vi "lib Hours Minutes Second to Degrees.vi"(8 "error in (no error)":errorcluster, 11 "Right Ascension cluster":T1) -> (0 "error out":errorcluster, 3 "Angle":dbl format="%#.8g")   [LabVIEW 2021]
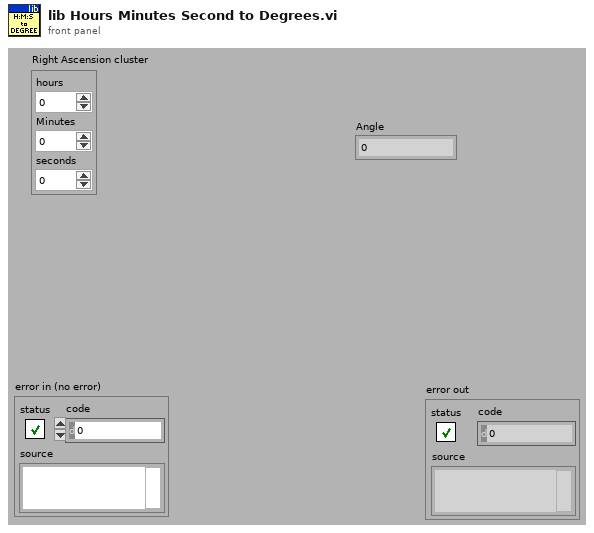
[diagram p1: front panel]
types:
  T1 = cluster{"hours":dbl, "Minutes":dbl, "seconds":dbl}
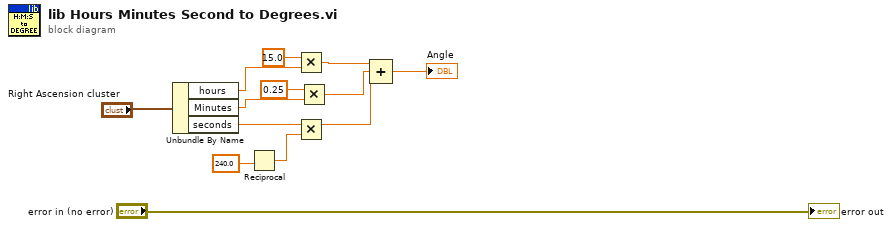
[diagram p0: block diagram]
diagram:
  n1 = Unbundle By Name("Right Ascension cluster") -> ("hours"=w11:dbl, "Minutes"=w9:dbl, "seconds"=w5:dbl)
  n2 = Reciprocal(x=240.0) -> (1/x=w1:dbl)
  n3 = Multiply(x=15.0, y=w11) -> (x*y=w7:dbl)
  n4 = Multiply(x=w5, y=w1) -> (x*y=w3:dbl)
  n5 = Multiply(x=0.25, y=w9) -> (x*y=w6:dbl)
  n6 = Compound Arithmetic op=ADD(w7, w6, w3) -> (→"Angle":dbl)
  "error out" <- "error in (no error)"
